vi "Shift Calculation.vi"(8 "error in (no error)":errorcluster, 9 "Current Time":timestamp, 10 "Time Stamp Out":timestamp[](array[timestamp])) -> (0 "error out":errorcluster, 2 "Shift":i32)   [LabVIEW 2023]
panel:
  in  "Shift Time Details":T1 {"3End" format="%<%H:%M:%S\n%x>T"; "2End" format="%<%H:%M:%S\n%x>T"; "3Start" format="%<%H:%M:%S\n%x>T"; "2Start" format="%<%H:%M:%S\n%x>T"; "1End" format="%<%H:%M:%S\n%x>T"; "1Start" format="%<%H:%M:%S\n%x>T"}
  # "Start Time"
  # "End Time"
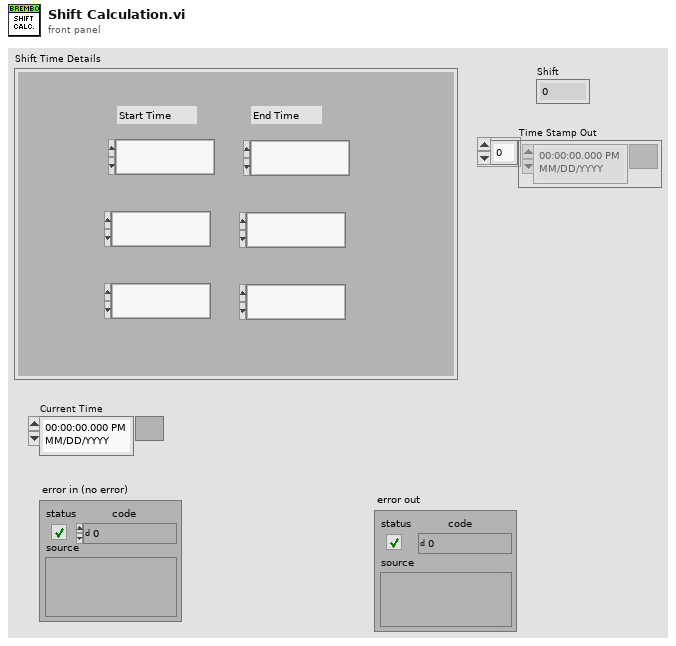
[diagram p1: front panel]
types:
  T1 = cluster{"1Start":timestamp, "1End":timestamp, "2Start":timestamp, "3Start":timestamp, "2End":timestamp, "3End":timestamp}
  T2 = typedef "LVDateTimeRec.ctl" = cluster{"fractional second":dbl, "second":i32, "minute":i32, "hour":i32, "day of month":i32, "month":i32, "year":i32, "day of week":i32, "day of year":i32, "DST":i32}
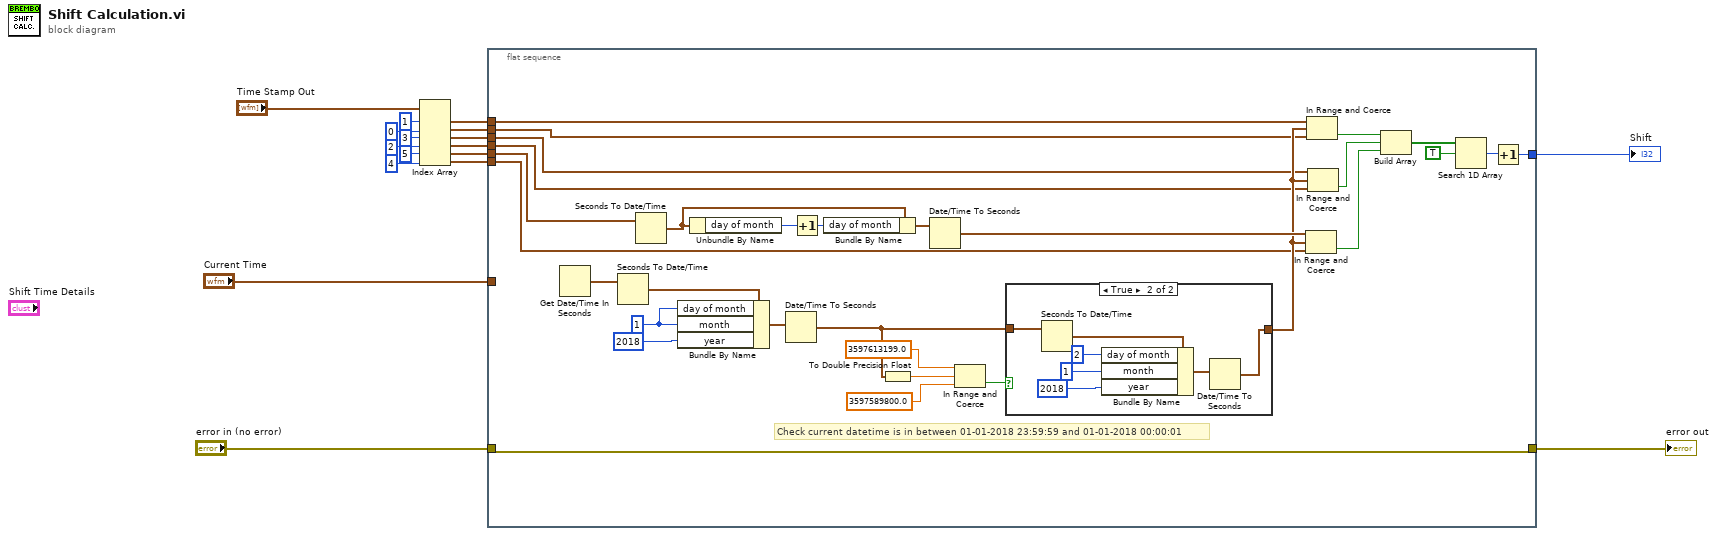
[diagram p0: block diagram]
diagram:
  n1 = Index Array(array="Time Stamp Out", index #1=1 ("index"), index #2=0 ("index"), index #3=3 ("index"), index #4=2 ("index"), index #5=5 ("index"), index #6=4 ("index")) -> (element #1=w10:timestamp, element #2=w9:timestamp, element #3=w6:timestamp, element #4=w5:timestamp, element #5=w2:timestamp, element #6=w1:timestamp)
  n2 = flat-sequence {
    tunnel: [w36] -> w17
    tunnel: "error in (no error)" -> [w25]
    tunnel: [w25] -> w15
    tunnel: "Current Time" -> [_]
    tunnel: w10 -> [w24]
    tunnel: w9 -> [w23]
    tunnel: w6 -> [w22]
    tunnel: w5 -> [w21]
    tunnel: w2 -> [w20]
    tunnel: w1 -> [w19]
    frame #0 {
      w29 = 1 ("day of month")
      # "Check current datetime is in between 01-01-2018 23:59:59 and 01-01-2018 00:00:01"
      n3 = Get Date/Time In Seconds() -> (seconds since 1Jan1904=w18:timestamp)
      n4 = Seconds To Date/Time(time stamp (now)=w18) -> (date time rec=w33:T2)  [unwired: 1 in]
      n5 = Seconds To Date/Time(time stamp (now)=w20) -> (date time rec=w46:T2)  [unwired: 1 in]
      n6 = Bundle By Name(cluster=w33, "day of month"=w29, "month"=w29, "year"=2018) -> (w35:T2)
      n7 = Unbundle By Name(w46) -> ("day of month"=w44:i32)
      n8 = Date/Time To Seconds(2:w35) -> (0:w27:timestamp)  [unwired: 1 in]
      n9 = Increment(x=w44) -> (x+1=w45:i32)
      n10 = Bundle By Name(cluster=w46, "day of month"=w45) -> (w47:T2)
      n11 = To Double Precision Float(number=w27) -> (double precision float=w30:dbl)
      n12 = Date/Time To Seconds(2:w47) -> (0:w43:timestamp)  [unwired: 1 in]
      n13 = In Range and Coerce(upper limit=3597613199.0 ("double precision float 2"), x=w30, lower limit=3597589800.0 ("double precision float")) -> (In Range?=w28:bool)  [unwired: 1 out]
      n14 = case shown="True" w28 {
        tunnel: w27 -> [w48 w51]
        tunnel: [w48 w50] -> w26
        frame False {
        }
        frame True {
          n15 = Seconds To Date/Time(time stamp (now)=w51) -> (date time rec=w53:T2)  [unwired: 1 in]
          n16 = Bundle By Name(cluster=w53, "day of month"=2, "month"=1 ("day of month"), "year"=2018) -> (w55:T2)
          n17 = Date/Time To Seconds(2:w55) -> (0:w50:timestamp)  [unwired: 1 in]
        }
      }
      n18 = In Range and Coerce(upper limit=w43, x=w26, lower limit=w19) -> (In Range?=w40:bool)  [unwired: 1 out]
      n19 = In Range and Coerce(upper limit=w24, x=w26, lower limit=w23) -> (In Range?=w42:bool)  [unwired: 1 out]
      n20 = In Range and Coerce(upper limit=w22, x=w26, lower limit=w21) -> (In Range?=w41:bool)  [unwired: 1 out]
      n21 = Build Array(w42, w41, w40) -> (w39:bool[])
      n22 = Search 1D Array(1D array=w39, element=TRUE) -> (index of element=w37:i32)  [unwired: 1 in]
      n23 = Increment(x=w37) -> (x+1=w36:i32)
    }
  }
  "Shift" <- w17
  "error out" <- w15
